vi "AutoDistanceGyro.vi"(1 "Reset Encoders":bool, 5 "TargetDistance":dbl, 7 "Motor Speed":dbl=0.8, 9 "InitialAngle":dbl, 11 "error in":errorcluster) -> (10 "InitialAngle Out":dbl, 15 "error out":errorcluster)   [LabVIEW 2012]
doc: "This VI is called when autonomous begins, and will automatically be terminated when autonomous ends. You can carry out timed or sensor driven robot movement independently without needing to return to the caller."
uses:
  <vilib>/Rock Robotics/WPI/RobotDrive/WPI_RobotDriveGetSetRefNum.vi
  <vilib>/addons/control/pid/pid.llb/PID (DBL).vi
  <vilib>/Rock Robotics/WPI/RobotDrive/WPI_RobotDriveArcadeDrive_Standard(NoSaturation).vi
  <vilib>/addons/control/pid/NI_PID_pid.lvlib
panel:
  in  "PID gains":T1={"proportional gain (Kc)"=0.05000000000000001, "integral time (Ti, min)"=0.006499999999999995, "derivative time (Td, min)"=0.001} {"proportional gain (Kc)" format="%_6g"; "integral time (Ti, min)" format="%_6g"; "derivative time (Td, min)" format="%_6g"}
  out "Distance (ft)":dbl
  out "OutputGraph":T2(graph)
  out "Current Angle":dbl
  out "Current Distance":dbl
  out "Angle Delta":dbl
  out "PID Output":dbl format="%.2f"
  # "Inputs"
  # "Outputs"
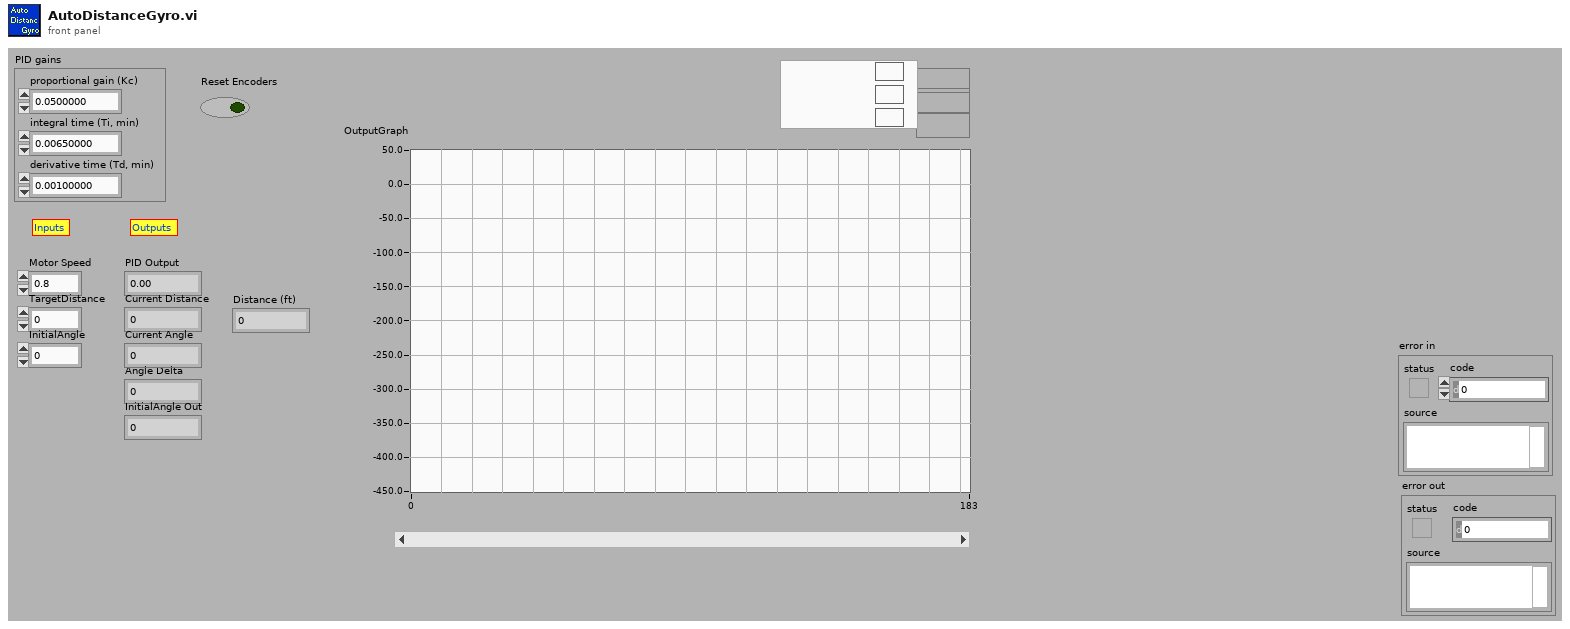
[diagram p1: front panel]
types:
  T1 = cluster{"proportional gain (Kc)":dbl, "integral time (Ti, min)":dbl, "derivative time (Td, min)":dbl}
  T2 = cluster{"Angle":dbl, "InitialAngle":dbl, "output":dbl}
  T3 = typedef "WPI_RobotDriveDevRef.ctl" = cluster{"DevStatus":errorcluster, "Motors[]":T4[], "Square Inputs":bool, "Max Output":dbl, "Isochronous":bool}
  T4 = typedef "WPI_MotorControlDeviceRef.ctl" = cluster{"DeviceStatus":errorcluster, "Type":enum16{"PWM", "CAN"}, "PWM":cluster{"Digital Module":T5, "PWM Channel":T6, "DeadBand":T7}, "CAN":cluster{"Device Number":u8, "Control Mode":T8, "Semaphore":T9, "Max Vout":dbl}, "Invert":bool, "TransformRef":T10, "InvTransformRef":T10}
  T5 = typedef "FPGA_TypedefDigitalModule.ctl" = enum16{"Digital Module 1", "Digital Module 2"}
  T6 = typedef "FPGA_DIOPWMChannel.ctl" = enum8{"PWM 1", "PWM 2", "PWM 3", "PWM 4", "PWM 5", "PWM 6", "PWM 7", "PWM 8", "PWM 9", "PWM 10", "Invalid"}
  T7 = typedef "WPI_PWMDeadband.ctl" = cluster{"Name":string, "maxPositivePwm":i32, "minPositivePwm":i32, "centerPwm":i32, "maxNegativePwm":i32, "minNegativePwm":i32, "angularRange":u16}
  T8 = typedef "WPI_CANJaguar_ControlMode.ctl" = enum8{"Percent VBus", "Current", "Speed", "Position", "Voltage"}
  T9 = typedef "Semaphore RefNum" = refnum<k1>
  T10 = typedef "WPI_PWMTransform_ConPane.ctl" = refnum<vi>
  T11 = typedef "WPI_GyroDevRef.ctl" = cluster{"DevStatus":errorcluster, "Analog Module":T12, "Analog Channel":T13, "Offset":dbl, "Gain (VoltsPerDegree/Second)":dbl}
  T12 = typedef "FPGA_TypedefAnalogModule.ctl" = enum16{"Analog Module 1", "Analog Module 2"}
  T13 = typedef "FPGA_AIChannel.ctl" = enum8{"AI 1", "AI 2", "AI 3", "AI 4", "AI 5", "AI 6", "AI 7", "AI 8", "Invalid"}
  T14 = cluster{"Output":dbl, "InitialAngle":dbl, "output":dbl}
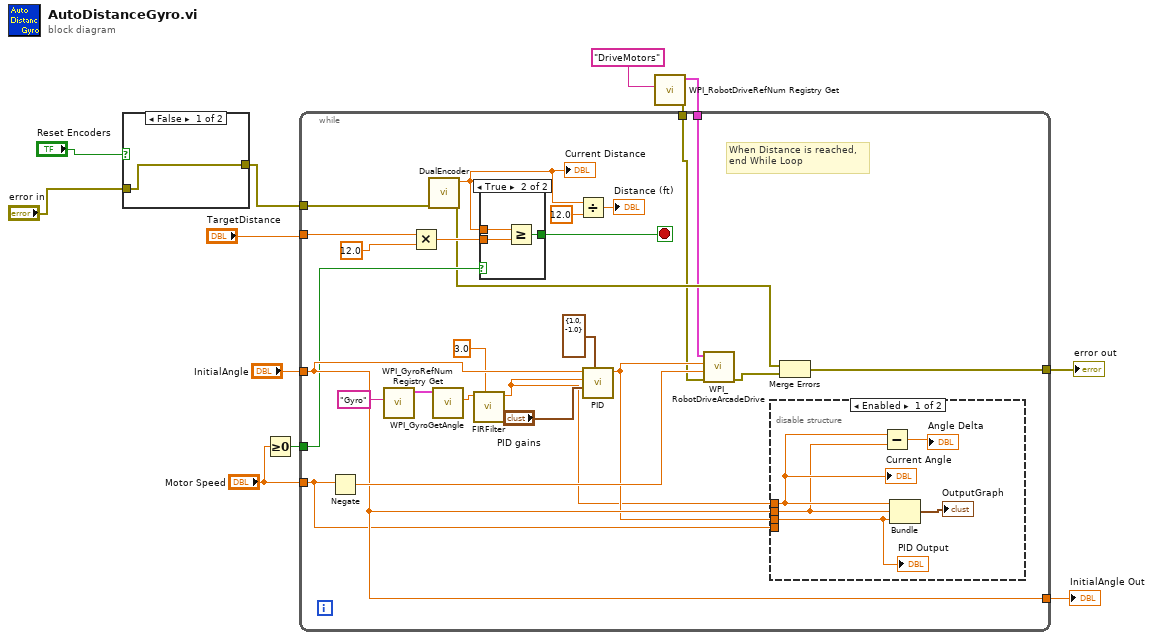
[diagram p0: block diagram]
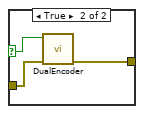
[diagram p2: hidden frame]
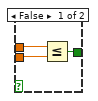
[diagram p3: hidden frame]
diagram:
  n1 = case shown="False" "Reset Encoders" {
    selector: "Reset Encoders" -> [_ w14]
    tunnel: "error in" -> [w13 w16]
    tunnel: [w13 w15] -> w2
    frame False {
    }
    frame True {
      n2 = call "DualEncoder.vi"("error in (no error)"=w16, "Reset?"=w14) -> ("error out"=w15:errorcluster)  [unwired: 6 in, 3 out]
    }
  }
  n3 = Greater Or Equal To 0?(x="Motor Speed") -> (x >= 0?=w9:bool)
  n4 = call <vilib>:"WPI_RobotDriveRefNum Registry Get.vi"("refnum name"="DriveMotors") -> ("error out"=w5:errorcluster, "RobotDriveDevRef"=w6:T3)  [unwired: 9 in]
  n5 = while {
    tunnel: "Motor Speed" -> [w36]
    tunnel: "TargetDistance" -> [w41]
    tunnel: "InitialAngle" -> [w37]
    tunnel: [w37] -> w10
    tunnel: w9 -> [w29]
    tunnel: [w25] -> w8
    tunnel: w2 -> [w26]
    tunnel: w6 -> [w24]
    tunnel: w5 -> [w22]
    stop <- w40 stop-if-true
    # "When Distance is reached, end While Loop"
    n6 = Negate(x=w36) -> (-x=w38:dbl)
    n7 = call <vilib>:"WPI_GyroRefNum Registry Get.vi"("refnum name"="Gyro") -> ("GyroDevRef"=w20:T11)  [unwired: 9 in, 1 out]
    n8 = Multiply(x=w41, y=12.0) -> (x*y=w30:dbl)
    n9 = call "DualEncoder.vi"("error in (no error)"=w26) -> ("error out"=w27:errorcluster, "Total Distance (in)"=w23:dbl)  [unwired: 7 in, 2 out]
    "Current Distance" <- w23
    n10 = call <vilib>:"WPI_GyroGetAngle.vi"("GyroDevRef"=w20) -> ("Angle"=w19:dbl)  [unwired: 1 in, 9 out]
    n11 = call "FIRFilter.vi"("Filter Size"=3.0, "Input"=w19) -> ("Output"=w18:dbl)  [unwired: 9 in]
    n12 = case shown="True" w29 {
      tunnel: [w44 w47] -> w40
      tunnel: w23 -> [w43 w46]
      tunnel: w30 -> [w42 w45]
      frame False {
        n13 = Less Or Equal?(x=w43, y=w42) -> (x <= y?=w44:bool)
      }
      frame True {
        n14 = Greater Or Equal?(x=w46, y=w45) -> (x >= y?=w47:bool)
      }
    }
    n15 = Divide(x=w23, y=12.0) -> (x/y=→"Distance (ft)":dbl)
    n16 = call-poly <vilib>:"PID.vi"("output range"=cluster{"output high":dbl, "output low":dbl} {"output high"=1.0, "output low"=-1.0}, "PID gains"="PID gains", "process variable"=w18, "setpoint"=w37) -> ("output"=w33:dbl)  [unwired: 2 in, 5 out]
    n17 = call-poly <vilib>:"WPI_RobotDriveArcadeDrive.vi"("error in (no error)"=w22, "Y axis value"=w38, "X axis value"=w33, "RobotDriveDevRef"=w24) -> ("error out"=w28:errorcluster)  [unwired: 5 in, 2 out]
    n18 = disable-structure shown="Enabled" {
      disable-tunnel: w18 -> [w49 _]
      disable-tunnel: w37 -> [w48 _]
      disable-tunnel: w36 -> [_ _]
      disable-tunnel: w33 -> [w51 _]
      frame Enabled {
        n19 = Subtract(x=w49, y=w48) -> (x-y=→"Angle Delta":dbl)
        n20 = Bundle("Output"=w49, "InitialAngle"=w48, "output"=w51) -> (→"OutputGraph":T14)  [unwired: 1 out]
        "PID Output" <- w51
        "Current Angle" <- w49
      }
      frame Disabled {
      }
    }
    n21 = Merge Errors(w27, w28) -> (w25:errorcluster)
  }
  "error out" <- w8
  "InitialAngle Out" <- w10
